vi "ChoiceNode_Create.vi"(0 "reference":refnum<class "ChoiceNode.lvclass">, 5 "error in (no error)":errorcluster) -> (14 "reference out":refnum<class "ChoiceNode.lvclass">, 19 "error out":errorcluster)   [LabVIEW 2020, in "ChoiceNode.lvclass"]
doc: "Creates and initializes a new StateNode object.\n\nThis object should be destroyed using a StateNode destructor VI or a virtual base class destructor VI.\n\n[GOOP 2.1]"
uses:
  <resource>/Framework/Providers/Open_GDS/UML/ChoiceNode_class/ChoiceNode.lvclass
  C:/Program Files (x86)/National Instruments/LabVIEW 2020/resource/Framework/Providers/Open_GDS/UML/RectangularNode_class/RectangularNode.lvclass
  <resource>/Framework/Providers/Open_GDS/UML/MultiLineString_class/SizeType.ctl
  <resource>/Framework/Providers/Open_GDS/UML/General/Rectangle/Rectangle Rectangle2D.ctl
  <resource>/Framework/Providers/Open_GDS/UML/MultiLineString_class/JustificationType.ctl
  <resource>/Framework/Providers/Open_GDS/UML/MultiLineString_class/MultiLineString.lvclass
  <resource>/Framework/Providers/Open_GDS/UML/RectangularNode_class/RectangularNode.lvclass
panel:
  # "The input reference should only\nbe wired when this method is called\nby a sub class constructor."
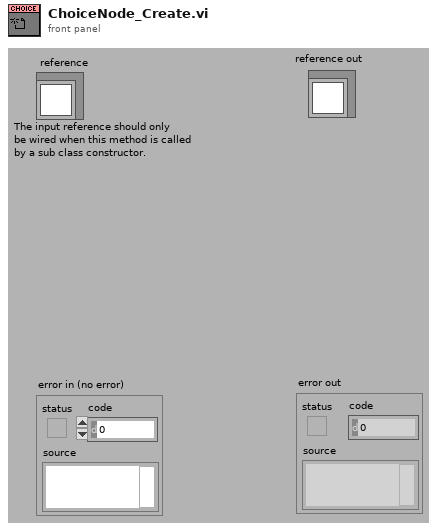
[diagram p1: front panel]
types:
  T1 = typedef "MultiLineString.lvclass/JustificationType.ctl" = enum16{"LEFT", "CENTER", "RIGHT"}
  T2 = typedef "Rectangle Rectangle2D.ctl" = cluster{"x":dbl, "y":dbl, "width":dbl, "height":dbl}
  T3 = typedef "MultiLineString.lvclass/SizeType.ctl" = enum16{"LARGE", "NORMAL", "SMALL"}
  T4 = typedef "ChoiceNode.lvclass/ObjectAttributes.ctl" = cluster{"Text":refnum<class "MultiLineString.lvclass">, "DEFAULT_WIDTH":i32, "DEFAULT_HEIGHT":i32}
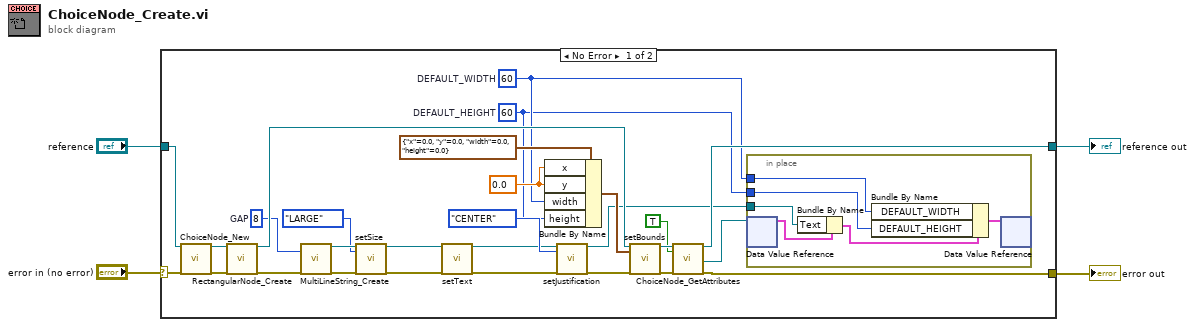
[diagram p0: block diagram]
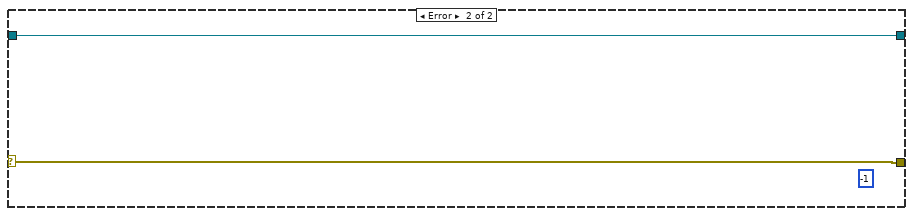
[diagram p2: hidden frame]
diagram:
  n1 = case shown="No Error" "error in (no error)" {
    selector: "error in (no error)" -> [w32 w40]
    tunnel: [w30 w39] -> w4
    tunnel: [w29 w40] -> w3
    tunnel: "reference" -> [w31 w39]
    frame No Error {
      w20 = 0.0 ("x")
      w12 = 8  # GAP
      w5 = 60  # DEFAULT_HEIGHT
      w6 = 60  # DEFAULT_WIDTH
      n2 = call <resource>:"ChoiceNode_New.vi"("reference in"=w31, "error in (no error)"=w32) -> ("reference out"=w19:refnum<class "ChoiceNode.lvclass">, "error out"=w28:errorcluster)  [unwired: 2 in, 14 out]
      n3 = call <resource>:"RectangularNode_Create.vi"("reference"=w19, "error in (no error)"=w28) -> ("reference out"=w23:refnum<class "ChoiceNode.lvclass">, "error out"=w13:errorcluster)  [unwired: 1 in, 15 out]
      n4 = call <resource>:"MultiLineString_Create.vi"("GAP"=w12, "error in (no error)"=w13) -> ("reference out"=w27:refnum<class "MultiLineString.lvclass">, "error out"=w26:errorcluster)  [unwired: 1 in, 15 out]
      n5 = call <resource>:"setSize.vi"("reference"=w27, "size"=SizeType."LARGE", "error in (no error)"=w26) -> ("reference out"=w17:refnum<class "MultiLineString.lvclass">, "error out"=w16:errorcluster)  [unwired: 15 out]
      n6 = call-dynamic "setText.vi"("reference"=w17, "error in (no error)"=w16) -> ("reference out"=w14:refnum<class "MultiLineString.lvclass">, "error out"=w15:errorcluster)  [unwired: 16 in]
      n7 = Bundle By Name(cluster=T2 {"x"=0.0, "y"=0.0, "width"=0.0, "height"=0.0} ("bounds"), "x"=w20, "y"=w20, "width"=w6, "height"=w5) -> (w22:T2)
      n8 = call <resource>:"setJustification.vi"("reference"=w14, "justification"=JustificationType."CENTER", "error in (no error)"=w15) -> ("reference out"=w7:refnum<class "MultiLineString.lvclass">, "error out"=w10:errorcluster)  [unwired: 15 out]
      n9 = call-dynamic "setBounds.vi"("reference"=w23, "bounds"=w22, "error in (no error)"=w10) -> ("reference out"=w11:refnum<class "ChoiceNode.lvclass">, "error out"=w18:errorcluster)  [unwired: 15 in]
      n10 = call <resource>:"ChoiceNode_GetAttributes.vi"("reference in"=w11, "OnlyGetDvrReference(False)"=TRUE, "error in (no error)"=w18) -> ("reference out"=w30:refnum<class "ChoiceNode.lvclass">, "DataRef"=w8:refnum<data-value>, "error out"=w29:errorcluster)  [unwired: 13 in, 1 out]
      n11 = in-place {
        in-place-border: w7 -> [w37]
        in-place-border: w6 -> [w35]
        in-place-border: w5 -> [w34]
        n12 = in-place-dvr #1(w8) -> (w38:T4)  [unwired: 1 out]
        n13 = Bundle By Name(cluster=w38, "Text"=w37) -> (w36:T4)
        n14 = Bundle By Name(cluster=w36, "DEFAULT_WIDTH"=w35, "DEFAULT_HEIGHT"=w34) -> (w33:T4)
        n15 = in-place-dvr #1(w33) -> ()  [unwired: 2 out]
      }
    }
    frame Error {
      (unwired) -1 ("Nr of open handles")
    }
  }
  "error out" <- w3
  "reference out" <- w4
